vi "read TBM configuration.vi"(8 "error in":errorcluster, 11 "CVT editor node in":refnum<class "TEC editor node.lvclass">) -> (0 "error out":errorcluster, 2 "configuration":refnum<class "TBM configuration.lvclass">, 3 "CVT editor node out":refnum<class "TEC editor node.lvclass">)   [LabVIEW 2013, in "TEC editor node.lvclass"]
uses:
  TEC editor node.lvclass
  <vilib>/NI/Tag Bus Module Framework/root configuration/TBM configuration.lvclass
  TEC editor node.lvclass/TEC editor node.ctl
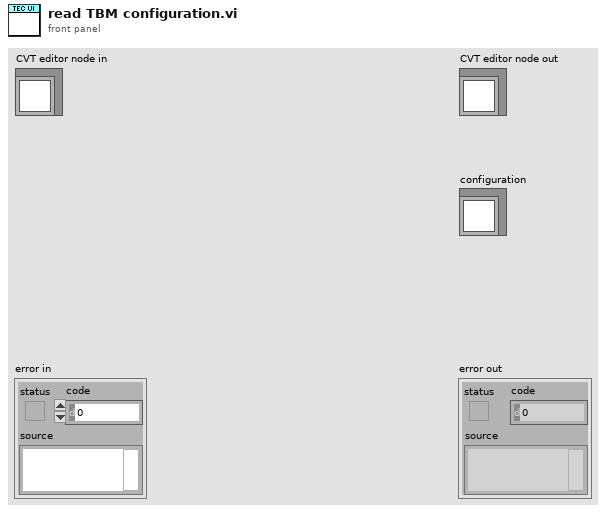
[diagram p1: front panel]
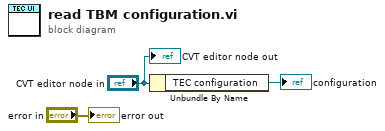
[diagram p0: block diagram]
diagram:
  n1 = Unbundle By Name("CVT editor node in") -> ("TEC configuration"=→"configuration":refnum<class "TEC configuration.lvclass">)
  "error out" <- "error in"
  "CVT editor node out" <- "CVT editor node in"
